vi "Client - Main.vi"(8 "error in (no error)":errorcluster) -> (0 "error out":errorcluster)   [LabVIEW 2019]
doc: "This VI should be run on the client PC."
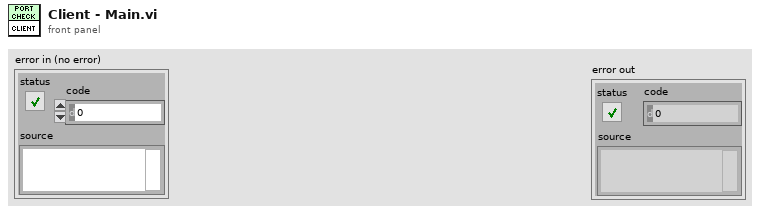
[diagram p1: front panel]
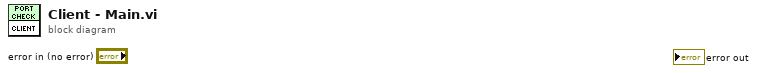
[diagram p0: block diagram]
diagram:
